vi "Test Basic.vi"(8 "error in":errorcluster) -> (0 "error out":errorcluster)   [LabVIEW 2013]
uses:
  <vilib>/addons/_JKI Toolkits/Caraya/classes/Test/Test.lvclass
  <vilib>/addons/_JKI Toolkits/Caraya/classes/Assert/Assert.lvclass
  source/Epochs -- enum.ctl
  <vilib>/addons/_JKI Toolkits/Caraya/classes/Assert/Assert True.vi
  <vilib>/addons/_JKI Toolkits/Caraya/classes/Assert/Assert False.vi
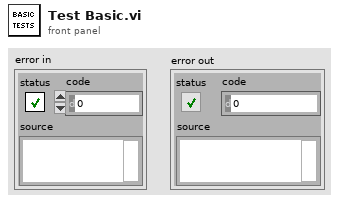
[diagram p1: front panel]
types:
  T1 = typedef "Epochs -- enum.ctl" = enum16{"Local", "UTC", "Unix", "GPS"}
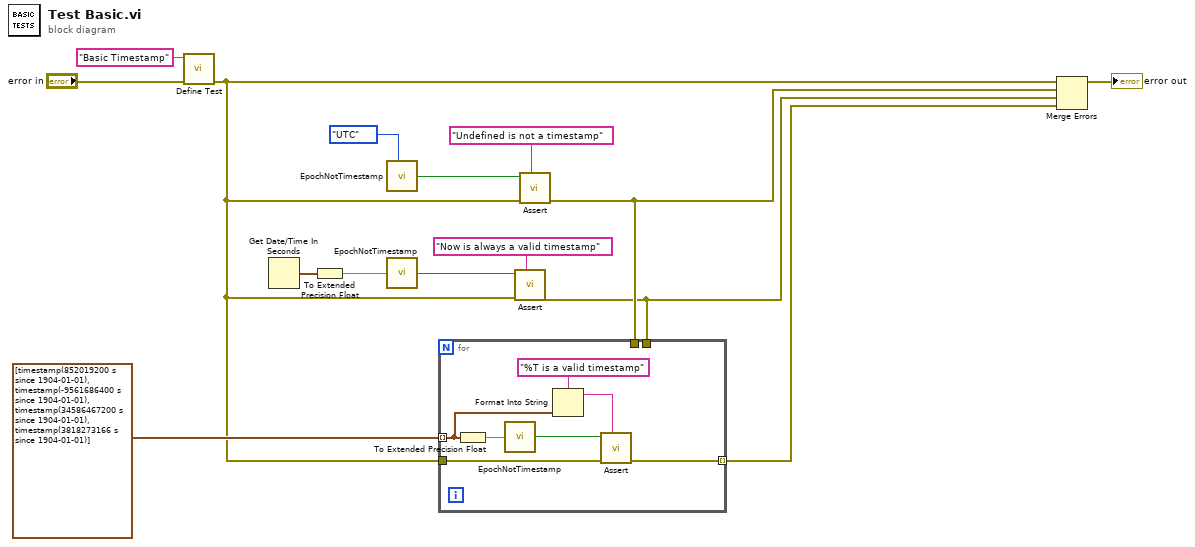
[diagram p0: block diagram]
diagram:
  n1 = call <vilib>:"Define Test.vi"("error in (no error)"="error in", "Label (VI Title)"="Basic Timestamp") -> ("error out"=w4:errorcluster)  [unwired: 8 in, 1 out]
  n2 = Get Date/Time In Seconds() -> (seconds since 1Jan1904=w8:timestamp)
  n3 = To Extended Precision Float(1:w8) -> (0:w9:ext)
  n4 = call "EpochNotTimestamp.vi"("Epoch (UTC)"=Epochs_--_enum."UTC") -> ("Not a Timestamp?"=w11:bool)  [unwired: 8 in]
  n5 = call "EpochNotTimestamp.vi"("Epoch Time"=w9) -> ("Not a Timestamp?"=w7:bool)  [unwired: 8 in]
  n6 = call-poly <vilib>:"Assert.vi"("Label"="Now is always a valid timestamp" ("Label (VI Title)"), "error in (no error)"=w4, "False?"=w7) -> ("error out"=w1:errorcluster)  [unwired: 7 in, 1 out]
  n7 = call-poly <vilib>:"Assert.vi"("Label"="Undefined is not a timestamp" ("Label (VI Title)"), "error in (no error)"=w4, "True?"=w11) -> ("error out"=w2:errorcluster)  [unwired: 7 in, 1 out]
  n8 = for {
    tunnel: timestamp[] [timestamp(852019200 s since 1904-01-01), timestamp(-9561686400 s since 1904-01-01), timestamp(34586467200 s since 1904-01-01), timestamp(3818273166.98601 s since 1904-01-01)] -> [w18] mode=indexing
    tunnel: w4 -> [w20]
    tunnel: [w19] -> w3 mode=indexing
    tunnel: w2 -> [_]
    tunnel: w1 -> [_]
    n9 = To Extended Precision Float(1:w18) -> (0:w22:ext)
    n10 = call "EpochNotTimestamp.vi"("Epoch Time"=w22) -> ("Not a Timestamp?"=w21:bool)  [unwired: 8 in]
    n11 = Format Into String(format string="%T is a valid timestamp" ("Label (VI Title)"), w18) -> (resulting string=w17:string)  [unwired: 2 in, 1 out]
    n12 = call-poly <vilib>:"Assert.vi"("Label"=w17, "error in (no error)"=w20, "False?"=w21) -> ("error out"=w19:errorcluster)  [unwired: 7 in, 1 out]
  }
  n13 = Merge Errors(w4, w2, w1, w3) -> (→"error out":errorcluster)
